vi "getFrontPanelRef.vi"(8 "error in (no error)":errorcluster, 11 "Rf_Ramp_Action in":refnum<class "Rf_Ramp_Action.lvclass">) -> (0 "error out":errorcluster, 2 "vi reference":refnum<vi>, 3 "Rf_Ramp_Action out":refnum<class "Rf_Ramp_Action.lvclass">)   [LabVIEW 2009, in "Views.lvlib" / "ScriptEditor.lvlib" / "Rf_Ramp_Action.lvclass"]
uses:
  Rf_Ramp_Action.lvclass
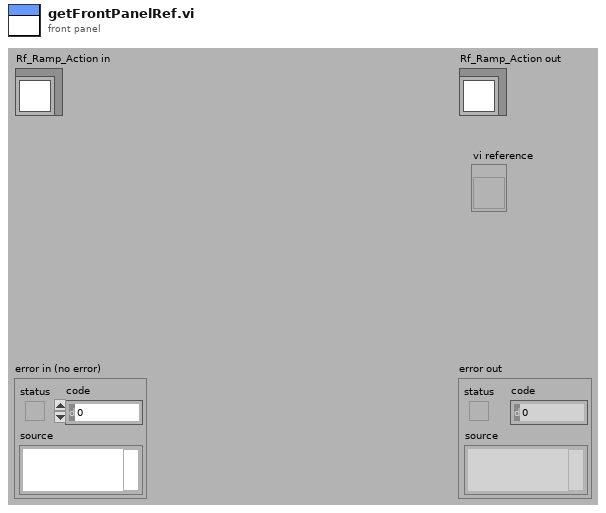
[diagram p1: front panel]
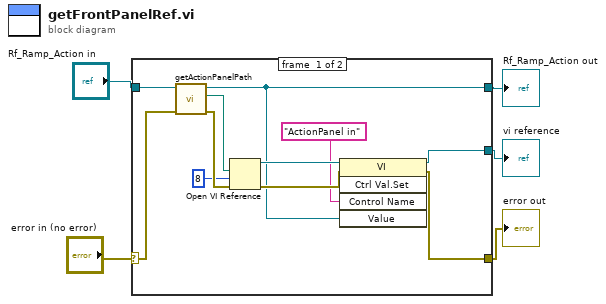
[diagram p0: block diagram]
diagram:
  n1 = case shown="No Error" "error in (no error)" {
    selector: "error in (no error)" -> [w15 w17]
    tunnel: "Rf_Ramp_Action in" -> [w16 w18]
    tunnel: [w6 w17] -> w2
    tunnel: [w9 w18] -> w3
    tunnel: [w7 _] -> w1
    frame #0 {
      n2 = call-dynamic "getActionPanelPath.vi"("error in (no error)"=w15, "Rf_Ramp_Action in"=w16) -> ("error out"=w13:errorcluster, "frontPanelPath"=w14:path, "Rf_Ramp_Action out"=w9:refnum<class "Rf_Ramp_Action.lvclass">)  [unwired: 7 in]
      n3 = Open VI Reference(vi path=w14, options=8, error in (no error)=w13) -> (vi reference=w11:refnum<vi>, error out=w10:errorcluster)  [unwired: 3 in]
      n4 = invoke class="VI" method="Ctrl Val.Set"(reference=w11, error in=w10, "Control Name"="ActionPanel in", "Value"=w9) -> (reference out=w7:refnum<vi>, error out=w6:errorcluster)  [unwired: 1 in, 3 out]
    }
    frame #1 {
    }
  }
  "error out" <- w2
  "Rf_Ramp_Action out" <- w3
  "vi reference" <- w1
